vi "Untitled 1.vi"() -> ()   [LabVIEW 2015]
panel:
  out "channel":string
  out "group":string
  out "String 2":string
  out "String":string
  in  "stop":bool
  in  "File contents":string(tree)
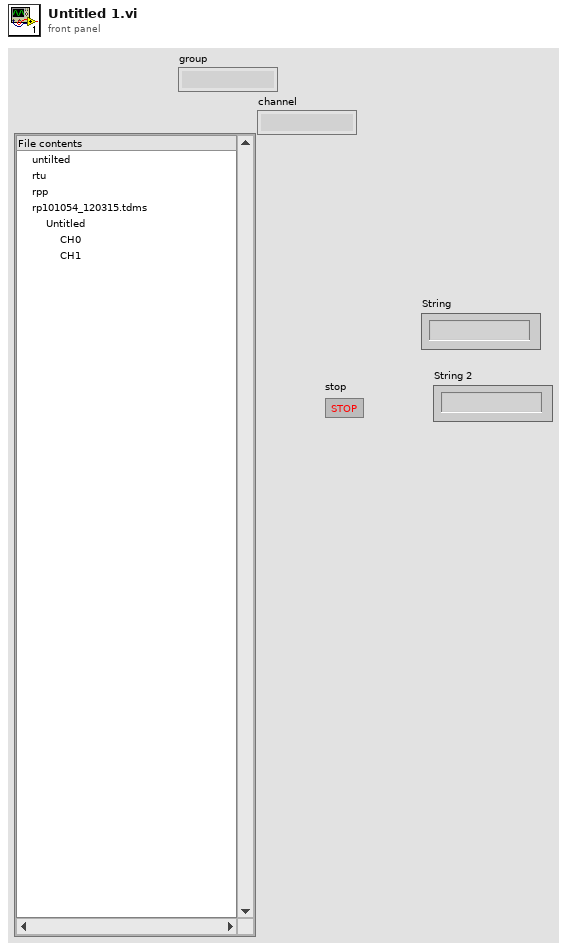
[diagram p1: front panel]
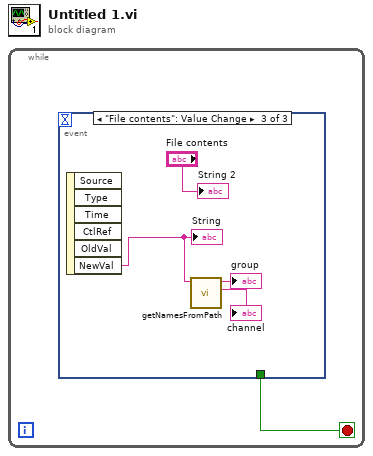
[diagram p0: block diagram]
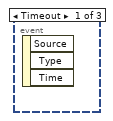
[diagram p2: hidden frame]
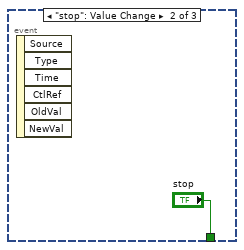
[diagram p3: hidden frame]
diagram:
  n1 = while {
    stop <- w1 stop-if-true
    n2 = event shown="[2] \"File contents\": Value Change" {
      selector: _ -> [_ _ _]
      dyn-events: _ -> [_ _ _]
      timeout: _ -> [_ _ _]
      tunnel: [_ "stop" _] -> w1
      event Timeout {
        n3 = event-data() -> ()  [unwired: 1 in, 3 out]
      }
      event "stop": Value Change {
        n4 = event-data() -> ()  [unwired: 1 in, 6 out]
      }
      event "File contents": Value Change {
        n5 = event-data() -> ("NewVal"=w5:string)  [unwired: 1 in, 5 out]
        "String" <- w5
        n6 = call "getNamesFromPath.vi"("tree path"=w5) -> ("channel"=→"channel":string, "group"=→"group":string)  [unwired: 2 in, 3 out]
        "String 2" <- "File contents"
      }
    }
  }
